vi "Vertical Scrollbar.vi"() -> ()   [LabVIEW 2023]
doc: "This VI demonstrates how to implement the user definable scrollbar control to add a scrolling feature to a cluster. \n\nThe feature is implemented by adjusting the coordinates of the controls and indicators in the cluster in relation to an increase or decrease of the scrollbar value."
panel:
  out "Cluster":T1={"Blue"=TRUE, "Green"=TRUE, "Yellow"=TRUE, "Red"=TRUE}
  in  "Stop":bool
  in  "Scrollbar":i32(c297)
  # "Overview: Demonstrates the use of the Vertical Scrollbar numeric control.\nInstructions:\n1. Run the VI.\n2. Adjust the scrollbar to view the items in the cluster.\n3. Click Stop to stop the VI."
  # "This is a cluster indicator that contains multiple LEDs outside its visible bounds. There is a Vertical Scrollbar control next to the cluster that can be used to programmatically change the viewing position of the contents of the cluster."
  # "Right-click the scrollbar and choose Properties, then select the Data Entry tab, to change its appearance."
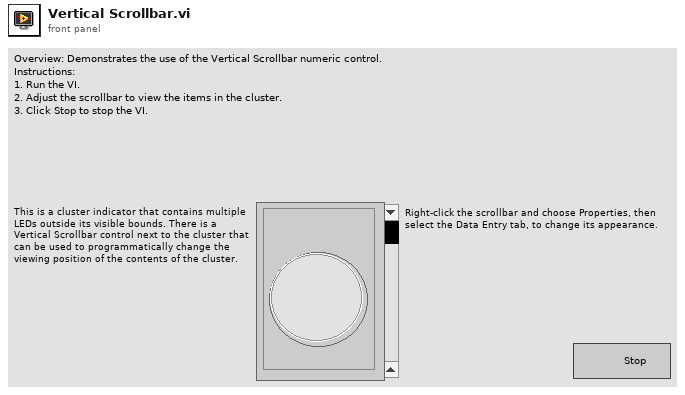
[diagram p1: front panel]
types:
  T1 = cluster{"Blue":bool, "Green":bool, "Yellow":bool, "Red":bool}
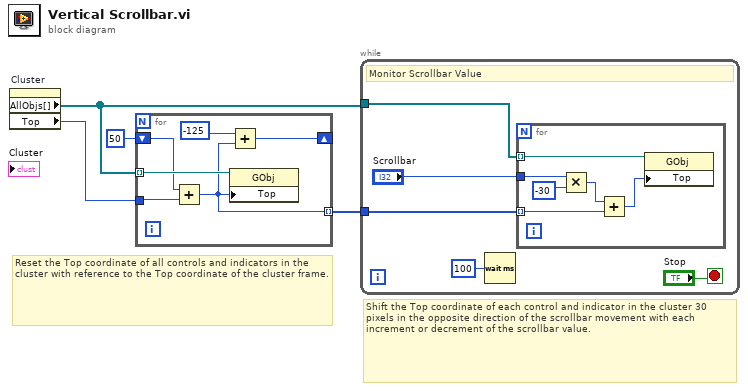
[diagram p0: block diagram]
diagram:
  # "Reset the Top coordinate of all controls and indicators in the cluster with reference to the Top coordinate of the cluster frame."
  # "Shift the Top coordinate of each control and indicator in the cluster 30 pixels in the opposite direction of the scrollbar movement with each increment or decrement of the scrollbar value."
  n1 = property on="Cluster" class="Clust (strict)"() -> ("AllObjs[]"=w2:refnum<vi>[], "Top"=w1:i32)  [unwired: 2 in, 2 out]
  n2 = for {
    tunnel: w2 -> [w10] mode=indexing
    tunnel: [w5] -> w4 mode=indexing
    shift-right: [w6] -> _
    shift-left: 50 -> [w9]
    tunnel: w1 -> [w8]
    n3 = Add(x=w9, y=w8) -> (x+y=w5:i32)
    n4 = Add(x=-125, y=w5) -> (x+y=w6:i32)
    n5 = property class="GObj"(reference=w10, "Top"=w5) -> ()  [unwired: 1 in, 2 out]
  }
  n6 = while {
    tunnel: w4 -> [w13]
    tunnel: w2 -> [w12]
    stop <- "Stop" stop-if-true
    # "Monitor Scrollbar Value"
    n7 = Wait (ms)(milliseconds to wait=u32 100) -> ()  [unwired: 1 out]
    n8 = for {
      tunnel: w12 -> [w20] mode=indexing
      tunnel: w13 -> [w21] mode=indexing
      tunnel: "Scrollbar" -> [w19]
      n9 = Multiply(x=w19, y=-30) -> (x*y=w18:i32)
      n10 = Add(x=w18, y=w21) -> (x+y=w17:i32)
      n11 = property class="GObj"(reference=w20, "Top"=w17) -> ()  [unwired: 1 in, 2 out]
    }
  }
